vi "test Create New Import Routing Channels.vi"(8 "error in (no error)":errorcluster, 11 "TestCase in":refnum<class "Routing and Faulting Import Unit Tests.lvclass">) -> (0 "error out":errorcluster, 3 "TestCase out":refnum<class "Routing and Faulting Import Unit Tests.lvclass">)   [LabVIEW 2020, in "Routing and Faulting Import Unit Tests.lvclass"]
uses:
  Routing and Faulting Import Unit Tests.lvclass
  Shared/Channel States.ctl
  Shared/Routing State.ctl
  Shared/Connection.ctl
  <vilib>/addons/_JKI Toolkits/VI Tester/TestCase.llb/TestCase.lvclass
  <vilib>/NI VeriStand/Custom Device Tools/Custom Device Utility Library/Custom Device Utility Library.lvlib
  Shared/Routing and Faulting Shared.lvlib
  Scripting/Routing and Faulting Scripting.lvlib
  C:/Program Files (x86)/National Instruments/LabVIEW 2020/vi.lib/addons/_JKI Toolkits/VI Tester/TestCase.llb/TestCase.lvclass
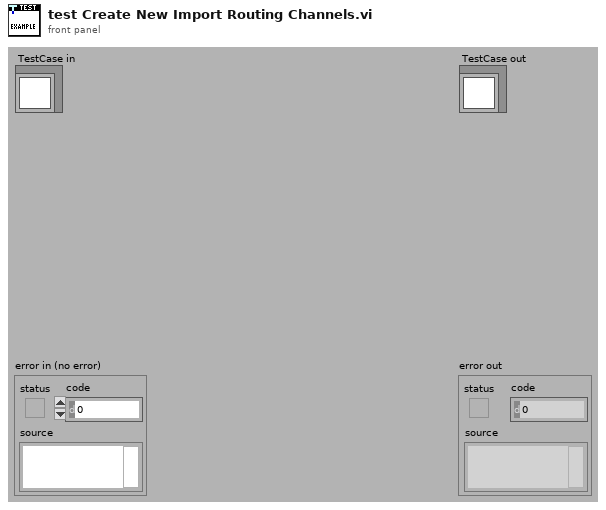
[diagram p1: front panel]
types:
  T1 = typedef "Routing and Faulting Shared.lvlib/Channel States.ctl" = T2[]
  T2 = typedef "Routing and Faulting Shared.lvlib/Routing State.ctl" = cluster{"Name":string, "Description":string, "Value":i32, "Connection List":T3[]}
  T3 = typedef "Routing and Faulting Shared.lvlib/Connection.ctl" = cluster{"Module":string, "Source":string, "Destination":string}
  T4 = cluster{"Channel Name":string, "Initial State":string, "Description":string, "State Configurations":T1}[]
  T5 = typedef "Custom Device API.lvlib/Custom Device Item Ref.ctl" = u64
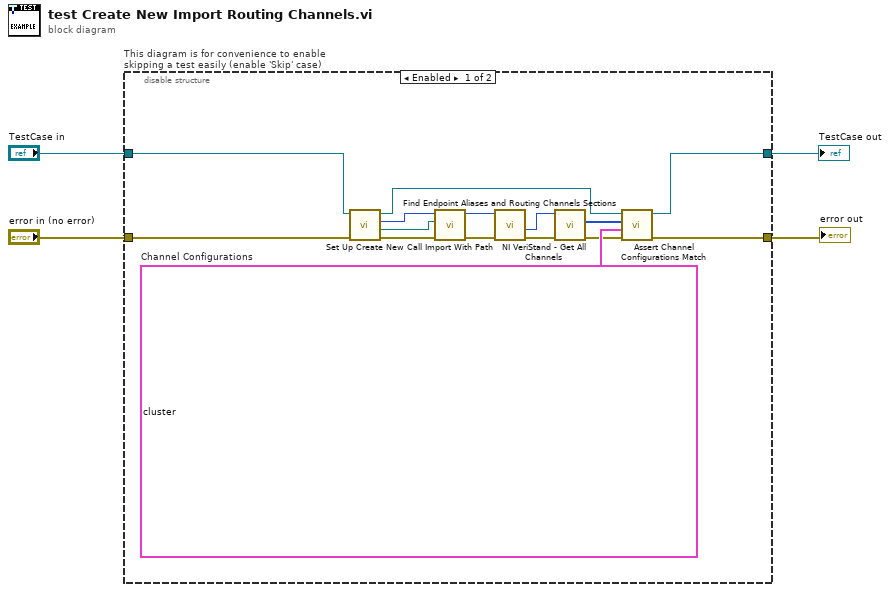
[diagram p0: block diagram]
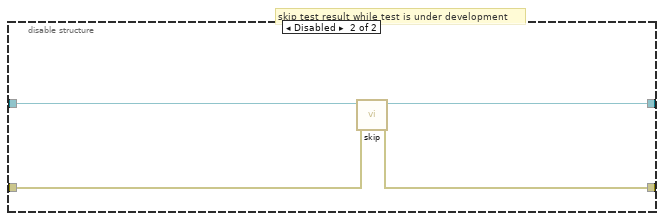
[diagram p2: hidden frame]
diagram:
  n1 = disable-structure "This diagram is for convenience to enable skipping a test easily (enable 'Skip' case)" shown="Enabled" {
    disable-tunnel: "TestCase in" -> [w15 w23]
    disable-tunnel: [w10 w21] -> w1
    disable-tunnel: [w11 w22] -> w3
    disable-tunnel: "error in (no error)" -> [w16 w20]
    frame Enabled {
      w13 = T4 [{"Channel Name"="Empty Channel", "Initial State"="No Connections", "Description"="Empty Channel", "State Configurations"=[{"Name"="No Connections", "Description"="State with no connections", "Value"=-1, "Connection List"=[]}]}, {"Channel Name"="Routing Channel", "Initial State"="One Connection", "Description"="This channel has some trivial states in it.", "State Configurations"=[{"Name"="No Connections", "Description"="State with no connections", "Value"=-1, "Connection List"=[]}, {"Name"="One Connection", "Description"="One connection in this state", "Value"=0, "Connection List"=[{"Module"="Targets/Controller/Hardware/SLSC/SLSC Chassis/Modules/Slot 2 (SLSC Switch)", "Source"="DUT_Ch0", "Destination"="LOAD_Ch0"}]}, {"Name"="Two Connections", "Description"="Two connections in this state", "Value"=10, "Connection List"=[{"Module"="Targets/Controller/Hardware/SLSC/SLSC Chassis/Modules/Slot 4 (SLSC Switch)", "Source"="DUT_Ch0", "Destination"="LOAD_Ch0"}, {"Module"="Targets/Controller/Hardware/SLSC/SLSC Chassis/Modules/Slot 2 (SLSC Switch)", "Source"="DUT_Ch0", "Destination"="LOAD_Ch0"}]}]}]  # Channel Configurations
      n2 = call "Set Up Create New.vi"("error in (no error)"=w16, "Test Case in"=w15) -> ("error out"=w14:errorcluster, "Import Path"=w8:path, "Routing and Faulting Custom Device Ref"=w7:T5, "Test Case out"=w9:refnum<class "Routing and Faulting Import Unit Tests.lvclass">)  [unwired: 6 in]
      n3 = call "Call Import With Path.vi"("error in (no error)"=w14, "Path"=w8, "Routing and Faulting Custom Device Ref in"=w7) -> ("error out"=w19:errorcluster, "Routing and Faulting Custom Device Ref out"=w6:T5)  [unwired: 7 in]
      n4 = call "Find Endpoint Aliases and Routing Channels Sections.vi"("error in"=w19, "routing and faulting custom device in"=w6) -> ("error out"=w18:errorcluster, "routing channels"=w17:T5)  [unwired: 6 in, 2 out]
      n5 = call <vilib>:"NI VeriStand - Get All Channels.vi"("error in"=w18, "Section Ref in"=w17) -> ("error out"=w12:errorcluster, "Channel Refs"=w5:T5[])  [unwired: 6 in, 2 out]
      n6 = call "Assert Channel Configurations Match.vi"("error in (no error)"=w12, "Channel Configurations"=w13, "Channel Refs"=w5, "Test Case in"=w9) -> ("error out"=w11:errorcluster, "Test Case out"=w10:refnum<class "Routing and Faulting Import Unit Tests.lvclass">)  [unwired: 6 in]
    }
    frame Disabled {
      # "skip test result while test is under development"
      n7 = call <vilib>:"skip.vi"("error in (no error)"=w20, "TestCase in"=w23) -> ("error out"=w22:errorcluster, "TestCase out"=w21:refnum<class "Routing and Faulting Import Unit Tests.lvclass">)  [unwired: 8 in]
    }
  }
  "error out" <- w3
  "TestCase out" <- w1
